vi "TDMS Write.vi"(7 "Channel Name":string, 8 "error in (no error)":errorcluster, 9 "Group Name":string, 10 "TDMS in":refnum<k34>, 11 "String Array in":refnum<class "String Array.lvclass">) -> (0 "error out":errorcluster, 2 "TDMS Out":refnum<k34>)   [LabVIEW 2020, in "Data.lvlib" / "String Array.lvclass"]
doc: "Write Generic Data to a TDMS file."
uses:
  String Array.lvclass
  String Array.lvclass/String Array.ctl
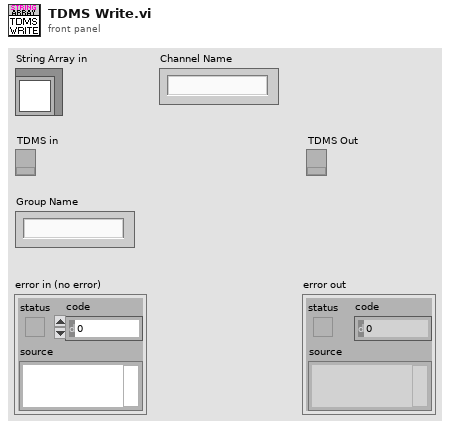
[diagram p1: front panel]
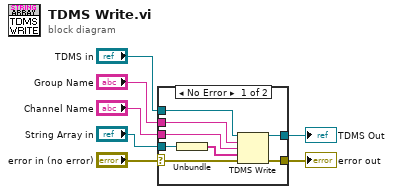
[diagram p0: block diagram]
diagram:
  n1 = case shown="No Error" "error in (no error)" {
    selector: "error in (no error)" -> [w15 w16]
    tunnel: [w14 w16] -> w6
    tunnel: "TDMS in" -> [w13 w17]
    tunnel: [w12 w17] -> w5
    tunnel: "Channel Name" -> [w11 _]
    tunnel: "Group Name" -> [w10 _]
    tunnel: "String Array in" -> [w9 _]
    frame No Error {
      n2 = Unbundle(w9) -> (w8:string[])
      n3 = TDMS Write(0:w13, 5:w10, 7:w11, 9:w8, 11:w15) -> (4:w12:refnum<k34>, 15:w14:errorcluster)  [unwired: 1 in, 2 out]
    }
    frame Error {
    }
  }
  "error out" <- w6
  "TDMS Out" <- w5
